vi "tcp combined test.vi"() -> ()   [LabVIEW 2015]
uses:
  communicator queue/identifying queue.lvclass
  client/connection client.lvclass/connection client.ctl
  communicator queue/identifying queue.lvclass/identifying queue.ctl
  message/communicator message.lvclass/communicator message.ctl
  client/prepare client.vi
  message/Read data.vi
  server/prepare server.vi
  message/set sender.vi
  TCP client/TCP client.lvclass
  TCP/TCP server.lvclass
  message/communicator message.lvclass
  communicator/communicator.lvclass
  connection/connection maintainer.lvclass
  <vilib>/ptbypt/NI_PtbyPt.lvlib
  manager/queue manager.lvclass
  communicator manager/communicator manager.lvlib
panel:
  out "ServQ":refnum<class "identifying queue.lvclass">
  out "ID 6":string
  out "data 6":variant
  out "ClienQ":refnum<class "identifying queue.lvclass">
  out "ID 5":string
  out "data 5":variant
  out "data 3":variant
  out "ID 3":string
  out "data":variant
  out "ID":string
  out "Numeric":dbl
  in  "Boolean":bool
  in  "remake s":bool
  in  "remake c":bool
  in  "CS 2":cluster{"ID":string, "data":string}
  in  "CS":cluster{"ID":string, "data":string}
  in  "S to C":bool
  in  "C to S":bool
  in  "exits":bool
  out "ClienT":timestamp
  out "servT":timestamp
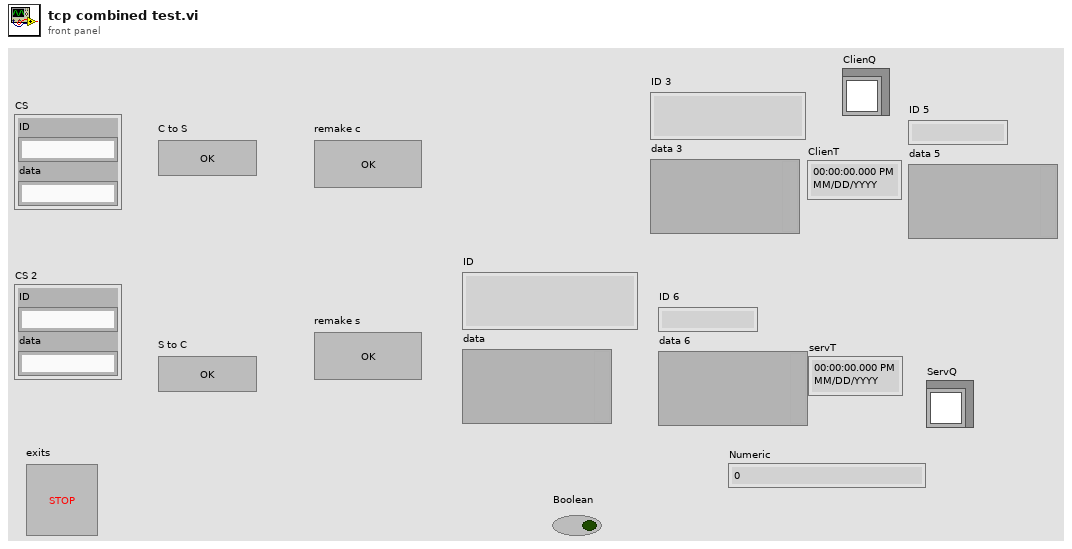
[diagram p1: front panel]
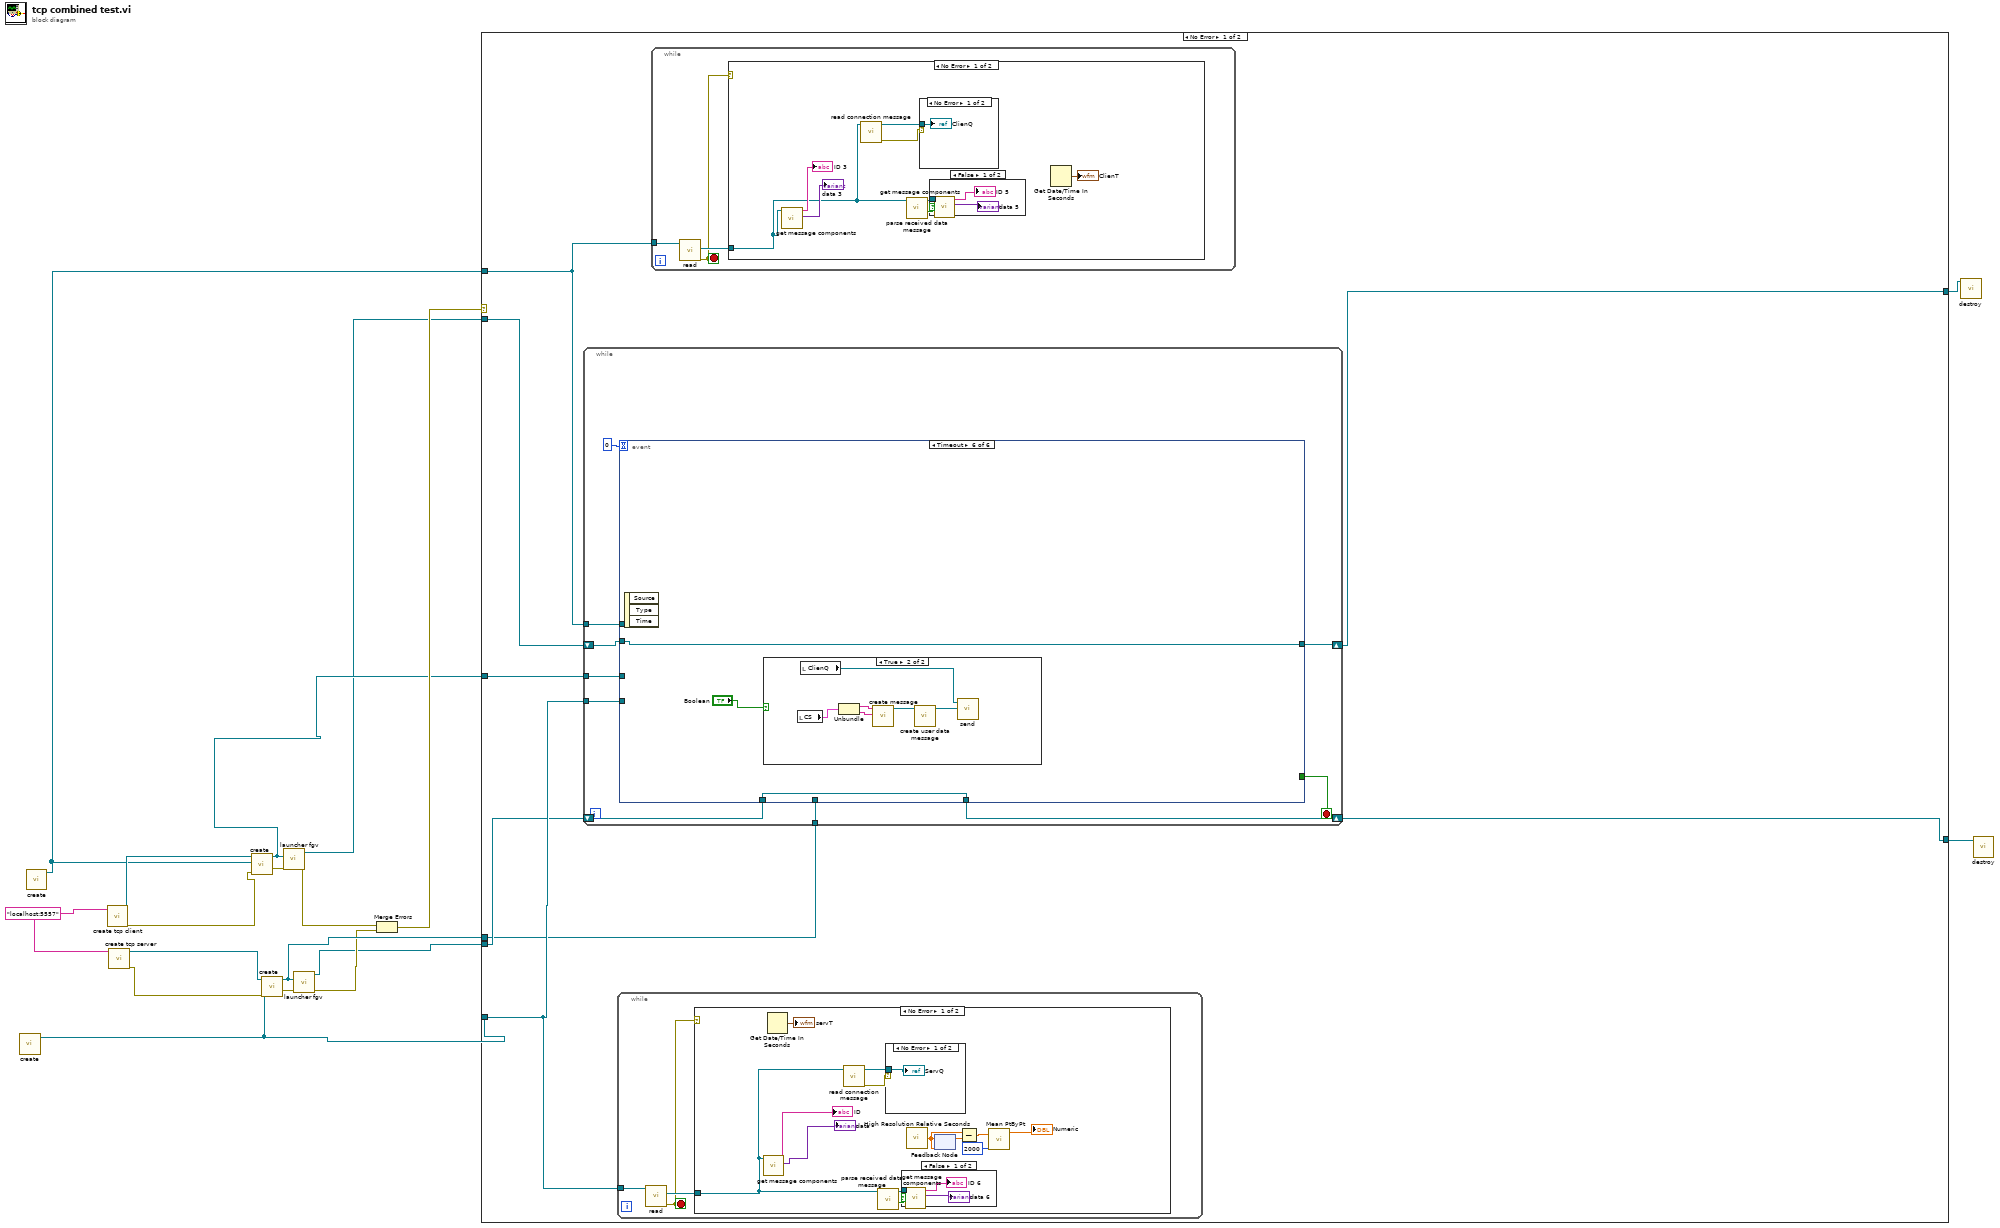
[diagram p0: block diagram]
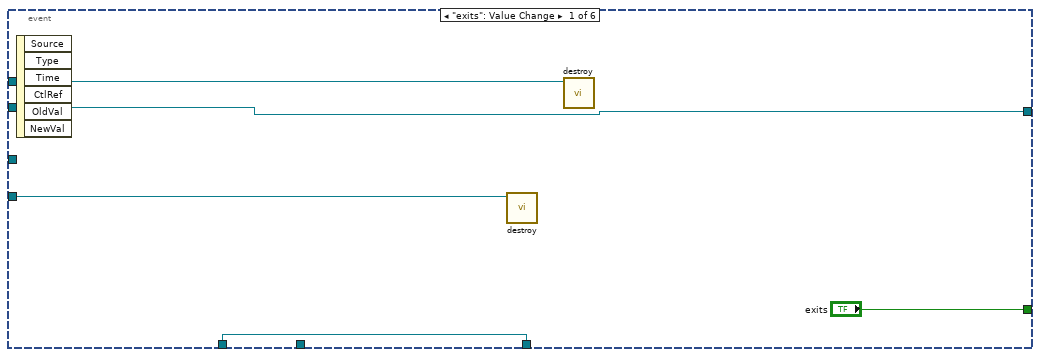
[diagram p2: hidden frame]
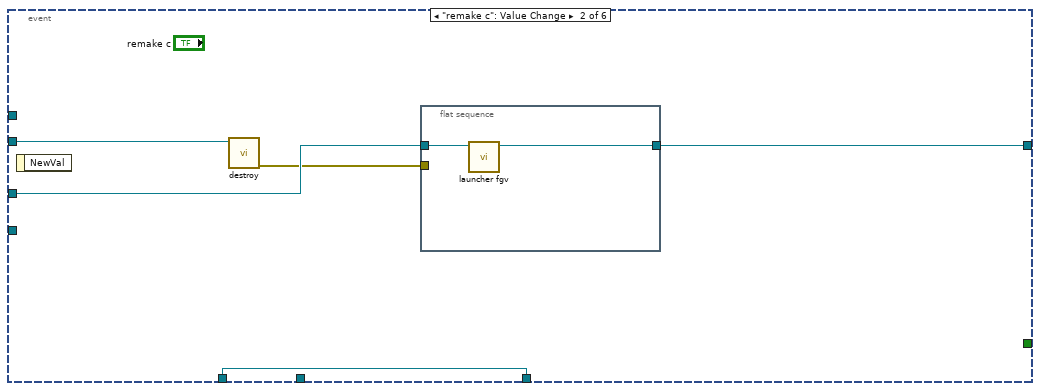
[diagram p3: hidden frame]
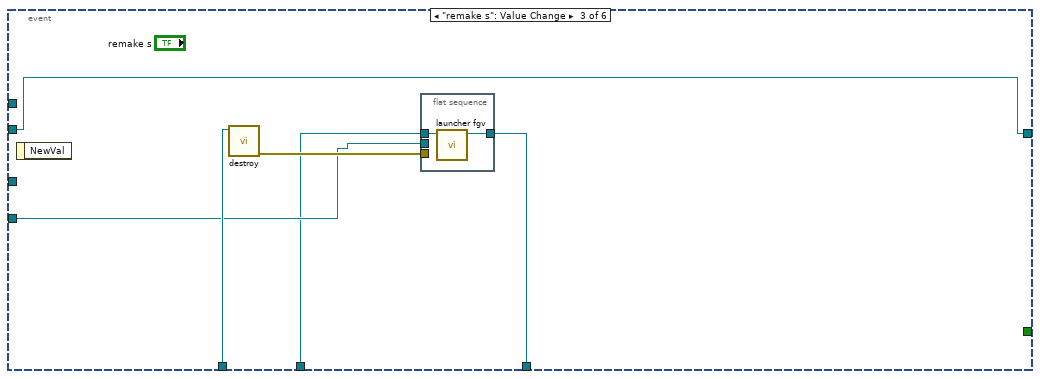
[diagram p4: hidden frame]
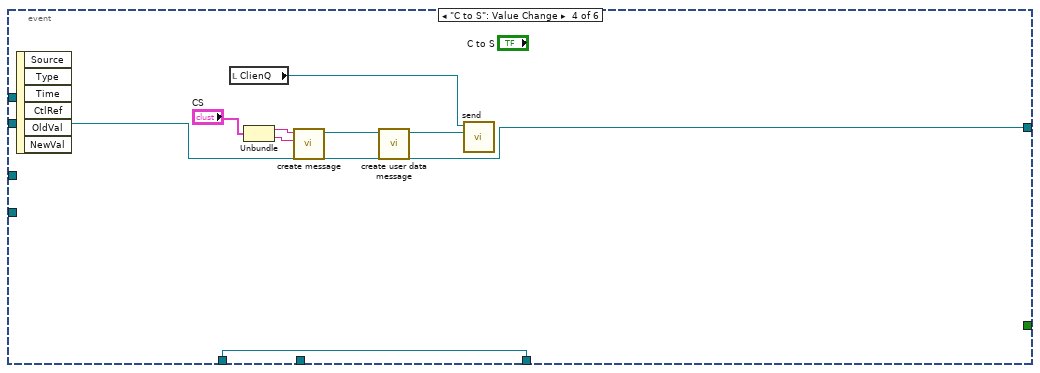
[diagram p5: hidden frame]
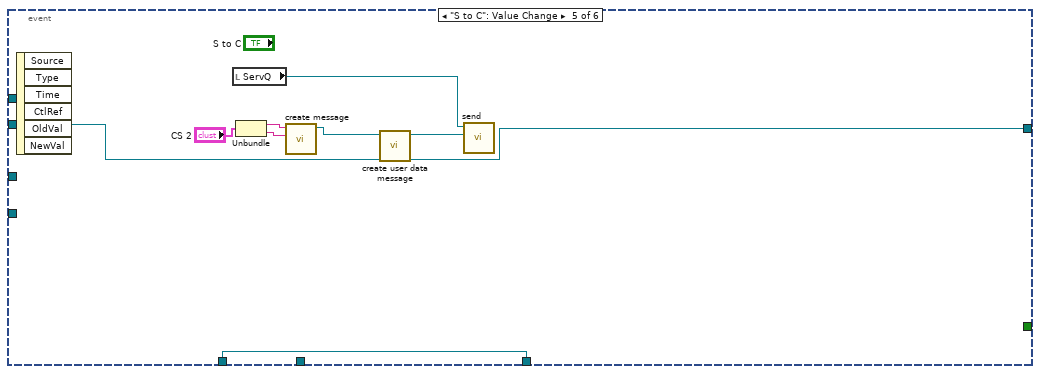
[diagram p6: hidden frame]
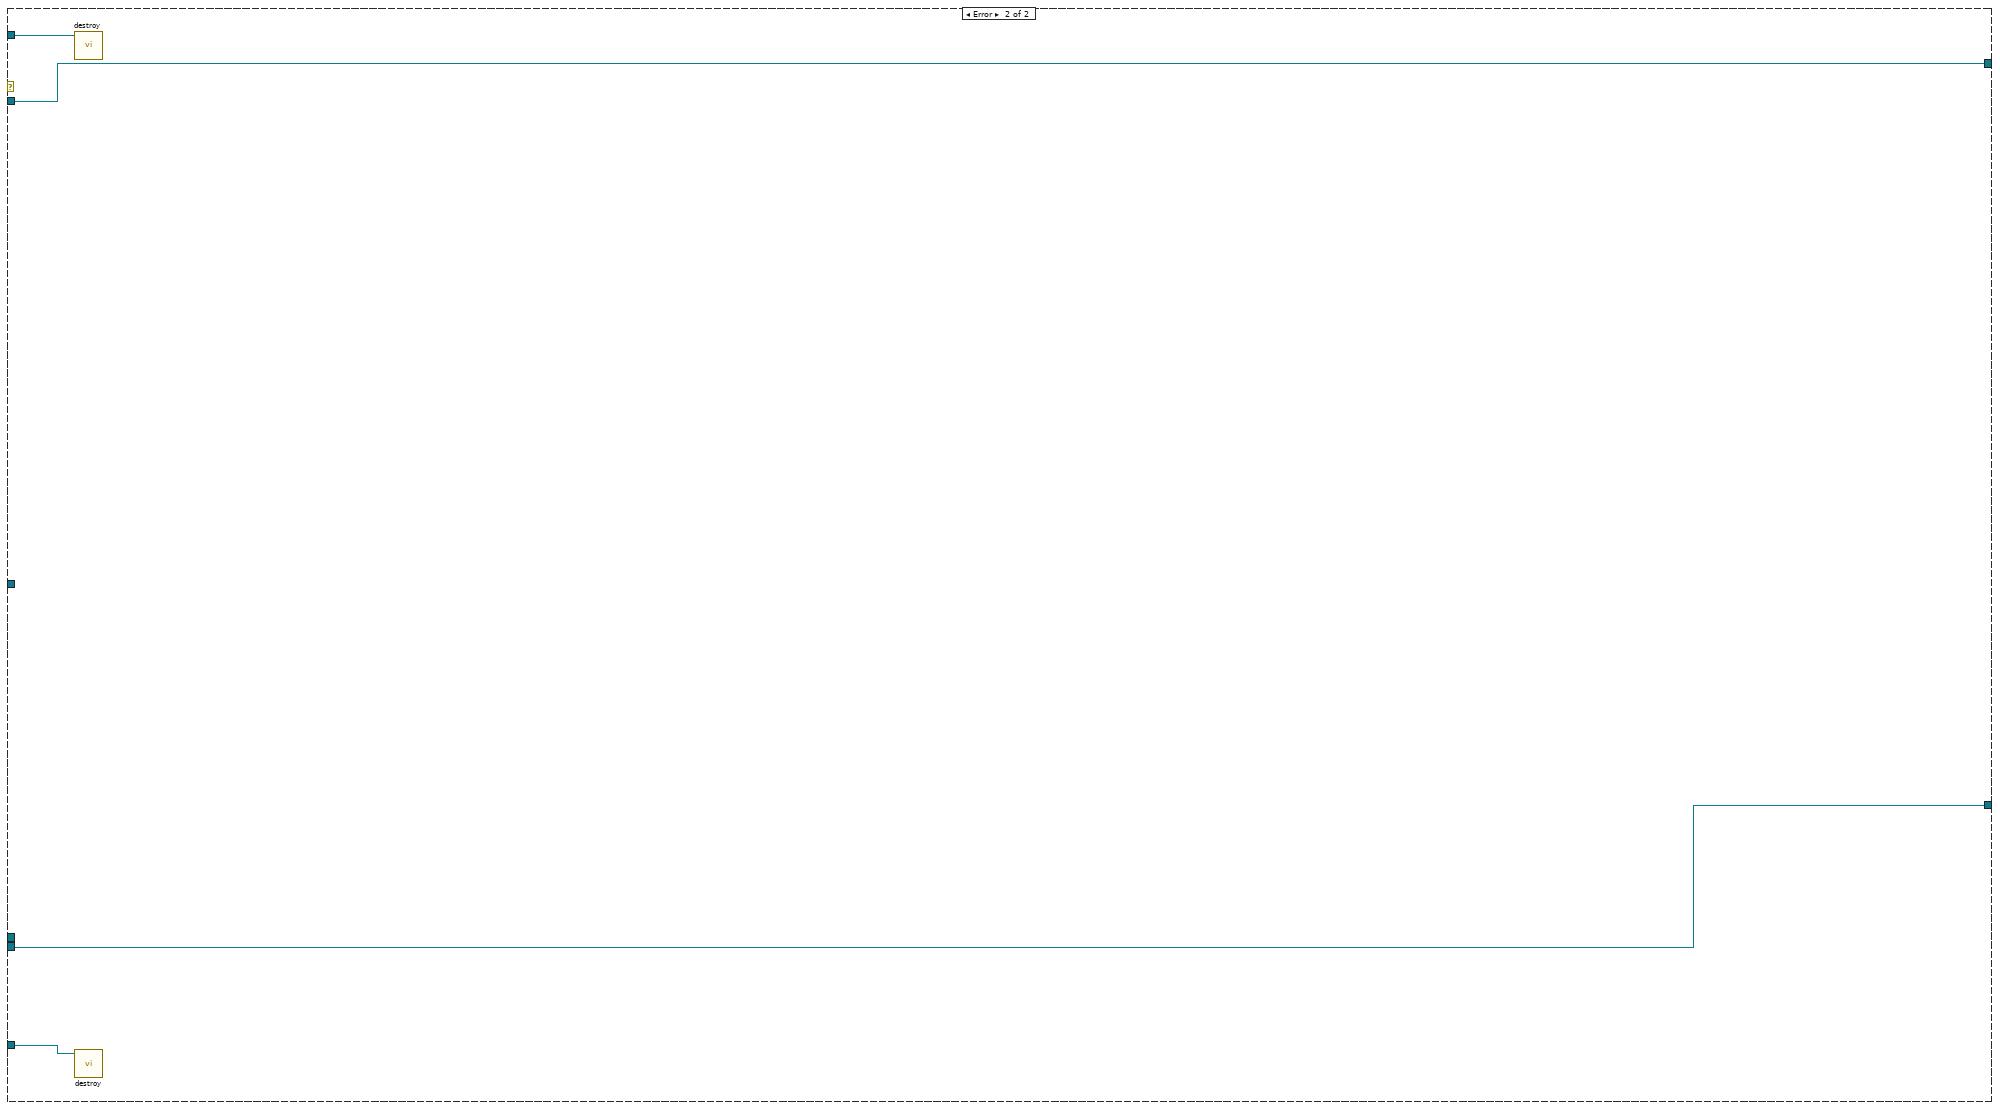
[diagram p14: hidden frame]
diagram:
  w17 = "localhost:5557" ("connection string")
  n1 = call "create.vi"() -> ("message connection out"=w1:refnum<class "identifying queue.lvclass">)  [unwired: 10 in, 1 out]
  n2 = call "create.vi"() -> ("message connection out"=w7:refnum<class "identifying queue.lvclass">)  [unwired: 10 in, 1 out]
  n3 = call "create tcp client.vi"("conn string"=w17) -> ("error out"=w9:errorcluster, "TCP client out"=w8:refnum<class "TCP client.lvclass">)  [unwired: 9 in]
  n4 = call "create tcp server.vi"("conn string"=w17) -> ("error out"=w4:errorcluster, "TCP server out"=w5:refnum<class "TCP server.lvclass">)  [unwired: 9 in]
  n5 = call "create.vi"("error in"=w9, "parent"=w7, "uninitialized communicator"=w8) -> ("error out"=w13:errorcluster, "communicator out"=w12:refnum<class "TCP client.lvclass">)  [unwired: 7 in]
  n6 = call "create.vi"("error in"=w4, "parent"=w1, "uninitialized communicator"=w5) -> ("error out"=w14:errorcluster, "communicator out"=w6:refnum<class "TCP server.lvclass">)  [unwired: 7 in]
  n7 = call "launcher fgv.vi"("error in"=w13, "communicator in"=w12) -> ("error out"=w10:errorcluster, "initialized communicator"=w11:refnum<class "communicator.lvclass">)  [unwired: 8 in]
  n8 = call "launcher fgv.vi"("error in"=w14, "communicator in"=w6) -> ("error out"=w3:errorcluster, "initialized communicator"=w2:refnum<class "communicator.lvclass">)  [unwired: 8 in]
  n9 = Merge Errors(w10, w3) -> (w16:errorcluster)
  n10 = case shown="No Error" w16 {
    tunnel: [w19 w119] -> w18
    tunnel: w7 -> [w25 w120]
    tunnel: w11 -> [w24 w119]
    tunnel: w1 -> [w26 w118]
    tunnel: w2 -> [w22 w117]
    tunnel: [w20 w117] -> w15
    tunnel: w12 -> [w23 _]
    tunnel: w6 -> [w21 _]
    frame No Error {
      n11 = while {
        tunnel: w26 -> [w35]
        tunnel: w25 -> [w34]
        tunnel: w23 -> [w32]
        tunnel: w21 -> [w30]
        shift-right: [w29] -> w20
        shift-left: w22 -> [w31]
        shift-right: [w28] -> w19
        shift-left: w24 -> [w33]
        stop <- w36 stop-if-true
        n12 = event shown="[5] Timeout" {
          selector: _ -> [_ _ _ _ _ _]
          dyn-events: _ -> [_ _ _ _ _ _]
          timeout: 0 -> [_ _ _ _ _ _]
          tunnel: ["exits" _ _ _ _ _] -> w36
          tunnel: w35 -> [w40 _ w52 _ _ _]
          tunnel: w34 -> [w39 _ _ _ _ _]
          tunnel: w33 -> [w37 w46 w49 w61 w69 w74]
          tunnel: w32 -> [_ w45 _ _ _ _]
          tunnel: w31 -> [w38 w43 w53 w62 w70 w75]
          tunnel: w30 -> [_ _ w51 _ _ _]
          tunnel: [w38 w43 w50 w62 w70 w75] -> w29
          tunnel: [w37 w42 w49 w61 w69 w74] -> w28
          event "exits": Value Change {
            n13 = event-data() -> ()  [unwired: 1 in, 6 out]
            n14 = call "destroy.vi"("message connection in"=w40) -> ()  [unwired: 10 in, 1 out]
            n15 = call "destroy.vi"("message connection in"=w39) -> ()  [unwired: 10 in, 1 out]
          }
          event "remake c": Value Change {
            n16 = event-data() -> ()  [unwired: 1 in, 1 out]
            n17 = call-dynamic "destroy.vi"("communicator in"=w46) -> ("error out"=w44:errorcluster)  [unwired: 10 in]
            n18 = flat-sequence {
              tunnel: w45 -> [w48]
              tunnel: w44 -> [_]
              tunnel: [w47] -> w42
              frame #0 {
                n19 = call "launcher fgv.vi"("communicator in"=w48) -> ("initialized communicator"=w47:refnum<class "communicator.lvclass">)  [unwired: 9 in, 1 out]
              }
            }
          }
          event "remake s": Value Change {
            n20 = event-data() -> ()  [unwired: 1 in, 1 out]
            n21 = call-dynamic "destroy.vi"("communicator in"=w53) -> ("error out"=w54:errorcluster)  [unwired: 10 in]
            n22 = flat-sequence {
              tunnel: w51 -> [w56]
              tunnel: w54 -> [_]
              tunnel: w52 -> [_]
              tunnel: [w55] -> w50
              frame #0 {
                n23 = call "launcher fgv.vi"("communicator in"=w56) -> ("initialized communicator"=w55:refnum<class "communicator.lvclass">)  [unwired: 9 in, 1 out]
              }
            }
          }
          event "C to S": Value Change {
            n24 = event-data() -> ()  [unwired: 1 in, 6 out]
            n25 = local read "ClienQ"() -> (w64:refnum<class "identifying queue.lvclass">)
            n26 = Unbundle("CS") -> ("ID"=w60:string, "data"=w59:string)
            n27 = call "create message.vi"("data"=w59, "ID"=w60) -> ("message"=w63:refnum<class "communicator message.lvclass">)  [unwired: 9 in]
            n28 = call "create user data message.vi"("data"=w63) -> ("message"=w57:refnum<class "communicator message.lvclass">)  [unwired: 10 in]
            n29 = call "send.vi"("message"=w57, "message connection in"=w64) -> ()  [unwired: 8 in, 2 out]
          }
          event "S to C": Value Change {
            n30 = event-data() -> ()  [unwired: 1 in, 6 out]
            n31 = local read "ServQ"() -> (w72:refnum<class "identifying queue.lvclass">)
            n32 = Unbundle("CS 2") -> ("ID"=w68:string, "data"=w67:string)
            n33 = call "create message.vi"("data"=w67, "ID"=w68) -> ("message"=w71:refnum<class "communicator message.lvclass">)  [unwired: 9 in]
            n34 = call "create user data message.vi"("data"=w71) -> ("message"=w65:refnum<class "communicator message.lvclass">)  [unwired: 10 in]
            n35 = call "send.vi"("message"=w65, "message connection in"=w72) -> ()  [unwired: 8 in, 2 out]
          }
          event Timeout {
            n36 = event-data() -> ()  [unwired: 1 in, 3 out]
            n37 = case shown="True" "Boolean" {
              frame False {
              }
              frame True {
                n38 = local read "CS"() -> (w79:cluster{"ID":string, "data":string})
                n39 = local read "ClienQ"() -> (w77:refnum<class "identifying queue.lvclass">)
                n40 = Unbundle(w79) -> ("ID"=w81:string, "data"=w80:string)
                n41 = call "create message.vi"("data"=w80, "ID"=w81) -> ("message"=w78:refnum<class "communicator message.lvclass">)  [unwired: 9 in]
                n42 = call "create user data message.vi"("data"=w78) -> ("message"=w76:refnum<class "communicator message.lvclass">)  [unwired: 10 in]
                n43 = call "send.vi"("message"=w76, "message connection in"=w77) -> ()  [unwired: 8 in, 2 out]
              }
            }
          }
        }
      }
      n44 = while {
        tunnel: w26 -> [w84]
        stop <- w82 stop-if-true
        n45 = call "read.vi"("identifying queue in"=w84) -> ("error out"=w82:errorcluster, "message"=w83:refnum<class "communicator message.lvclass">)  [unwired: 8 in, 1 out]
        n46 = case shown="No Error" w82 {
          tunnel: w83 -> [w85 _]
          frame No Error {
            n47 = call "get message components.vi"("message"=w85) -> ("data"=→"data":variant, "ID"=→"ID":string)  [unwired: 9 in]
            n48 = Get Date/Time In Seconds() -> (seconds since 1Jan1904=→"servT":timestamp)
            n49 = call "read connection message.vi"("communicator message in"=w85) -> ("error out"=w96:errorcluster, "queue"=w97:refnum<class "identifying queue.lvclass">)  [unwired: 9 in]
            n50 = call "parse received data message.vi"("message"=w85) -> ("invalid?"=w86:bool, "data"=w87:refnum<class "communicator message.lvclass">)  [unwired: 9 in]
            n51 = case shown="No Error" w96 {
              tunnel: w97 -> [w101 _]
              frame No Error {
                "ServQ" <- w101
              }
              frame Error {
              }
            }
            n52 = case shown="False" w86 {
              tunnel: w87 -> [w100 _]
              frame False {
                n53 = call "get message components.vi"("message"=w100) -> ("data"=→"data 6":variant, "ID"=→"ID 6":string)  [unwired: 9 in]
              }
              frame True {
              }
            }
            n54 = call <vilib>:"High Resolution Relative Seconds.vi"() -> ("relative seconds"=w93:dbl)
            n55 = feedback-in #1(w93) -> ()
            n56 = feedback #1(w93) -> (w94:dbl)
            n57 = Subtract(x=w93, y=w94) -> (x-y=w92:dbl)
            n58 = call <vilib>:"Mean PtByPt.vi"("x"=w92, "sample length"=2000) -> ("mean"=→"Numeric":dbl)  [unwired: 2 in, 1 out]
          }
          frame Error {
          }
        }
      }
      n59 = while {
        tunnel: w25 -> [w104]
        stop <- w102 stop-if-true
        n60 = call "read.vi"("identifying queue in"=w104) -> ("error out"=w102:errorcluster, "message"=w103:refnum<class "communicator message.lvclass">)  [unwired: 8 in, 1 out]
        n61 = case shown="No Error" w102 {
          tunnel: w103 -> [w105 _]
          frame No Error {
            n62 = call "get message components.vi"("message"=w105) -> ("data"=→"data 3":variant, "ID"=→"ID 3":string)  [unwired: 9 in]
            n63 = call "read connection message.vi"("communicator message in"=w105) -> ("error out"=w111:errorcluster, "queue"=w112:refnum<class "identifying queue.lvclass">)  [unwired: 9 in]
            n64 = call "parse received data message.vi"("message"=w105) -> ("invalid?"=w106:bool, "data"=w107:refnum<class "communicator message.lvclass">)  [unwired: 9 in]
            n65 = case shown="No Error" w111 {
              tunnel: w112 -> [w116 _]
              frame No Error {
                "ClienQ" <- w116
              }
              frame Error {
              }
            }
            n66 = case shown="False" w106 {
              tunnel: w107 -> [w115 _]
              frame False {
                n67 = call "get message components.vi"("message"=w115) -> ("data"=→"data 5":variant, "ID"=→"ID 5":string)  [unwired: 9 in]
              }
              frame True {
              }
            }
            n68 = Get Date/Time In Seconds() -> (seconds since 1Jan1904=→"ClienT":timestamp)
          }
          frame Error {
          }
        }
      }
    }
    frame Error {
      n69 = call "destroy.vi"("message connection in"=w120) -> ()  [unwired: 10 in, 1 out]
      n70 = call "destroy.vi"("message connection in"=w118) -> ()  [unwired: 10 in, 1 out]
    }
  }
  n71 = call-dynamic "destroy.vi"("communicator in"=w18) -> ()  [unwired: 10 in, 1 out]
  n72 = call-dynamic "destroy.vi"("communicator in"=w15) -> ()  [unwired: 10 in, 1 out]
